vi "BELLA_iPhone_server.vi"() -> ()   [LabVIEW 2013]
uses:
  VIremote.llb/VIremoteFunction.ctl
panel:
  in  "stopmain":bool
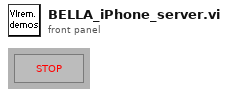
[diagram p1: front panel]
types:
  T1 = typedef "VIremoteInit.ctl" = cluster{"port (2055)":u16, "Use mouse emulation (T)":bool, "Use keyboard emulation (T)":bool, "Allow multiple connections (F)":bool, "Debug mode/error dialog (F)":bool, "Temporary directory (default)":path, "Mouse emulation VI path":path, "Keyboard emulation VI path":path, "Enable VI Select button(T)":bool, "Enable auto scroll(T)":bool}
  T2 = typedef "VIremoteFunction.ctl" = enum16{"Do nothing", "Stop controller", "Close this connection", "Show info panel", "Set VI to control", "Set Accelerometer freq (Hz)", "Show Alert message", "Start Sound Input", "Stop Sound Input", "Set Volume (0-100)", "Set sound output Speaker", "Set sound output Receiver", "Play Sound", "Repeat Sound", "Stop Sound", "Pause Sound", "Resume Sound", "Set panel width of caller (320 or 480)", "Set Panel Size to Portrait", "Set Panel Size to Landscape", "Set Panel Size as Current Orientation", "Allow all UI Orientations", "Send user notification", "Disable Scrolling", "Normal Scrolling", "Page Scrolling", "Set Scroll Offset", "Page Indicator Position"}
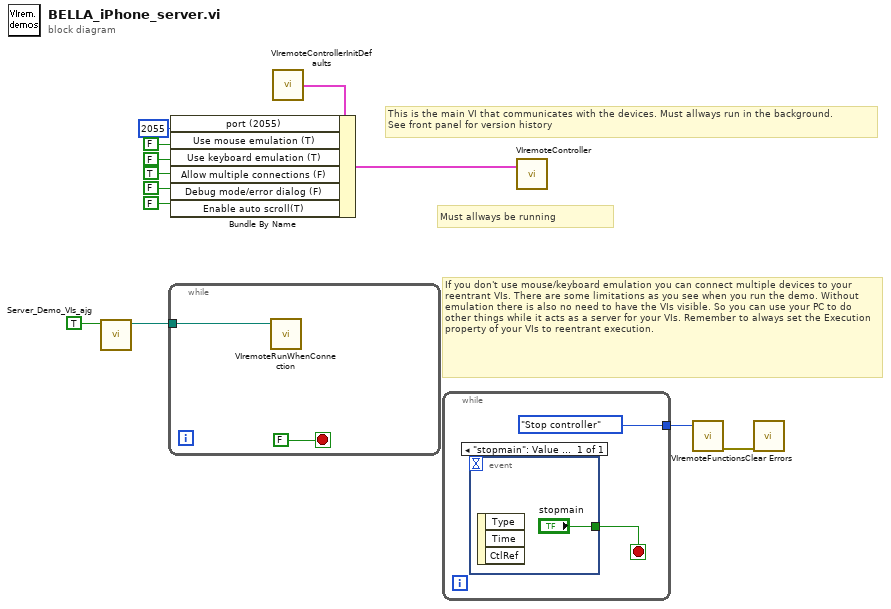
[diagram p0: block diagram]
diagram:
  # "If you don't use mouse/keyboard emulation you can connect multiple devices to your reentrant VIs. There are some limitations as you see when you run the demo. Without emulation there is also no need to have the VIs visible. So you can use your PC to do other things while it acts as a server for your VIs. Remember to always set the Execution property of your VIs to reentrant execution."
  # "Must allways be running"
  # "This is the main VI that communicates with the devices. Must allways run in the background.\nSee front panel for version history"
  n1 = call "Server_Demo_VIs_ajg.vi"("Only get This VIs path"=TRUE) -> ("path"=w12:path)  [unwired: 10 in]
  n2 = while {
    tunnel: w12 -> [w13]
    stop <- FALSE stop-if-true
    n3 = call "VIremoteRunWhenConnection.vi"("path to VI that will be run"=w13) -> ()  [unwired: 1 in, 10 out]
  }
  n4 = call "VIremoteControllerInitDefaults.vi"() -> ("Init defaults"=w3:T1)
  n5 = Bundle By Name(cluster=w3, "port (2055)"=u16 2055, "Use mouse emulation (T)"=FALSE, "Use keyboard emulation (T)"=FALSE, "Allow multiple connections (F)"=TRUE, "Debug mode/error dialog (F)"=FALSE, "Enable auto scroll(T)"=FALSE) -> (w11:T1)
  n6 = while {
    tunnel: [VIremoteFunction."Stop controller" ("Function")] -> w6
    stop <- w16 stop-if-true
    n7 = event shown="[0] \"stopmain\": Value Change" {
      selector: _ -> [_]
      dyn-events: _ -> [_]
      timeout: _ -> [_]
      tunnel: ["stopmain"] -> w16
      event "stopmain": Value Change {
        n8 = event-data() -> ()  [unwired: 4 out]
      }
    }
  }
  n9 = call "VIremoteController.vi"("Init (can't be changed while running)"=w11) -> ()  [unwired: 11 out]
  n10 = call "VIremoteFunctions.vi"("Function"=w6) -> ("error out"=w1:errorcluster)  [unwired: 5 in, 5 out]
  n11 = call <vilib>:"Clear Errors.vi"("error in (no error)"=w1) -> ()  [unwired: 6 in, 1 out]
